vi "Calculate Ramp Displacements.vi"(1 "Iterative\nRamp":bool, 2 "LBCB Selected":T3, 3 "Ramp Time":dbl) -> (0 "Target":T1)   [LabVIEW 2009]
uses:
  Data Access Objects/Metadata/LBCB Number.ctl
  Target Data.ctl
  Data Access Objects/Metadata/LBCB Space.ctl
  Data Access Objects/Metadata/DAO Actions.ctl
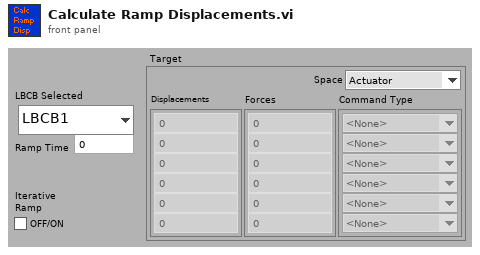
[diagram p1: front panel]
types:
  T1 = typedef "Target Data.ctl" = cluster{"Displacements":dbl[], "Command Type":enum16{"<None>", "Displacement", "Force"}[], "Forces":dbl[], "Space":T2}
  T2 = typedef "LBCB Space.ctl" = enum16{"Actuator", "Cartesian"}
  T3 = typedef "LBCB Number.ctl" = enum16{"LBCB1", "LBCB2"}
  T4 = typedef "DAO Actions.ctl" = enum16{"Init", "Get", "Set"}
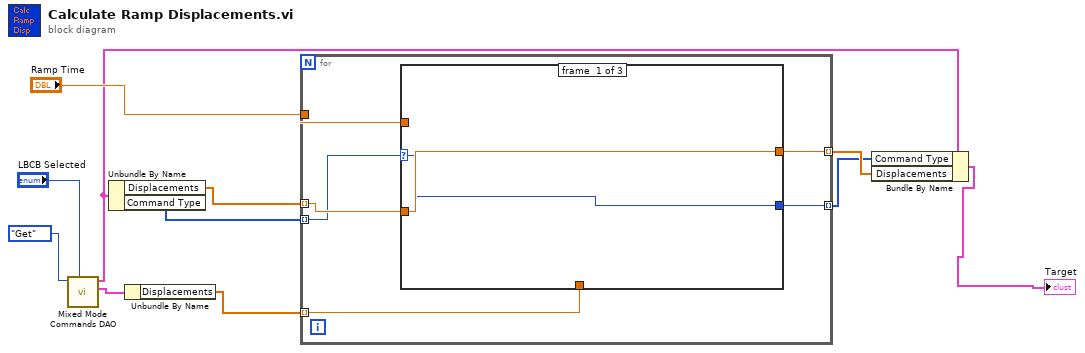
[diagram p0: block diagram]
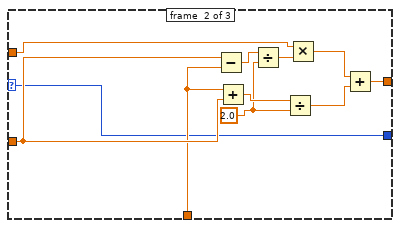
[diagram p2: hidden frame]
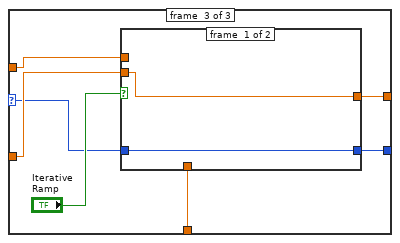
[diagram p3: hidden frame]
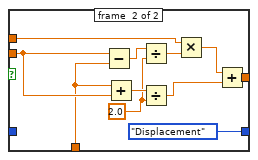
[diagram p4: hidden frame]
diagram:
  n1 = call "Mixed Mode Commands DAO.vi"("LBCB Selected"="LBCB Selected", "Mixed Mode Commands\n Datastore Actions"=DAO_Actions."Get" ("Mixed Mode Commands\n Datastore Actions")) -> ("Previous Target"=w9:T1, "Current Target"=w6:T1)  [unwired: 3 in, 5 out]
  n2 = Unbundle By Name(w6) -> ("Displacements"=w10:dbl[], "Command Type"=w7:enum16{"<None>", "Displacement", "Force"}[])
  n3 = Unbundle By Name(w9) -> ("Displacements"=w8:dbl[])
  n4 = for {
    tunnel: w10 -> [w17] mode=indexing
    tunnel: w8 -> [w16] mode=indexing
    tunnel: [w15] -> w5 mode=indexing
    tunnel: "Ramp Time" -> [w14]
    tunnel: w7 -> [w13] mode=indexing
    tunnel: [w12] -> w3 mode=indexing
    n5 = case shown="\"Displacement\"" w13 {
      selector: w13 -> [w18 w20 w31]
      tunnel: w17 -> [w19 w30 w37]
      tunnel: w16 -> [_ w29 w36]
      tunnel: [w19 w28 w35] -> w15
      tunnel: w14 -> [_ w27 w34]
      tunnel: [w18 w20 w32] -> w12
      frame #0 {
      }
      frame #1 {
        w24 = 2.0 ("y")
        n6 = Subtract(x=w30, y=w29) -> (x-y=w25:dbl)
        n7 = Add(x=w29, y=w30) -> (x+y=w26:dbl)
        n8 = Divide(x=w25, y=w24) -> (x/y=w23:dbl)
        n9 = Divide(x=w26, y=w24) -> (x/y=w21:dbl)
        n10 = Multiply(x=w27, y=w23) -> (x*y=w22:dbl)
        n11 = Add(x=w22, y=w21) -> (x+y=w28:dbl)
      }
      frame #2 {
        n12 = case shown="False" "Iterative\nRamp" {
          tunnel: w37 -> [w39 w50]
          tunnel: w36 -> [_ w49]
          tunnel: [w39 w48] -> w35
          tunnel: w34 -> [_ w47]
          tunnel: [w38 enum16{"<None>", "Displacement", "Force"}."Displacement" ("Enum")] -> w32
          tunnel: w31 -> [w38 _]
          frame #0 {
          }
          frame #1 {
            w44 = 2.0 ("y")
            n13 = Subtract(x=w50, y=w49) -> (x-y=w45:dbl)
            n14 = Add(x=w49, y=w50) -> (x+y=w46:dbl)
            n15 = Divide(x=w45, y=w44) -> (x/y=w43:dbl)
            n16 = Divide(x=w46, y=w44) -> (x/y=w41:dbl)
            n17 = Multiply(x=w47, y=w43) -> (x*y=w42:dbl)
            n18 = Add(x=w42, y=w41) -> (x+y=w48:dbl)
          }
        }
      }
    }
  }
  n19 = Bundle By Name(cluster=w6, "Command Type"=w3, "Displacements"=w5) -> (→"Target":T1)
